vi "CIPC Universal FIFO.vi"() -> (3 "CIF_CIPC_Universal.lvclass":refnum<class "CIF_CIPC_Universal.lvclass">)   [LabVIEW 2021, in "CIF_CIPC_Universal.lvclass"]
uses:
  CIF_CIPC_Universal.lvclass
  CIF_CIPC_Universal.lvclass/CIF_CIPC_Universal.ctl
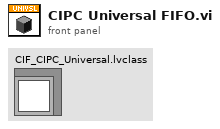
[diagram p1: front panel]
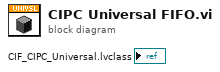
[diagram p0: block diagram]
diagram:
